vi "DIFFERENT OPERATIONS ON VALUES.vi"() -> ()   [LabVIEW 2015]
panel:
  in  "CHOOSE THE OPERATION":T1(ring)
  out "OUTPUT":dbl
  in  "NUM 2":dbl
  in  "NUM 1":dbl
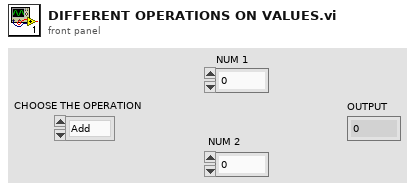
[diagram p1: front panel]
types:
  T1 = enum16{"Add", "Subtract", "Multiply", "Divide", "Max", "Min", "square", "sqrt", "avg"}
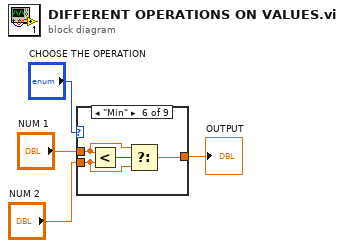
[diagram p0: block diagram]
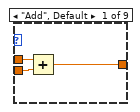
[diagram p2: hidden frame]
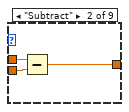
[diagram p3: hidden frame]
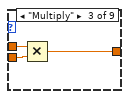
[diagram p4: hidden frame]
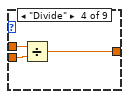
[diagram p5: hidden frame]
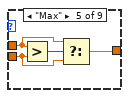
[diagram p6: hidden frame]
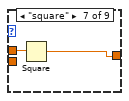
[diagram p7: hidden frame]
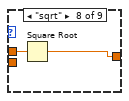
[diagram p8: hidden frame]
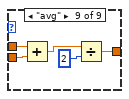
[diagram p9: hidden frame]
diagram:
  n1 = case shown="\"Min\"" "CHOOSE THE OPERATION" {
    tunnel: "NUM 1" -> [w7 w10 w13 w16 w19 w22 w26 w28 w33]
    tunnel: "NUM 2" -> [w6 w9 w12 w15 w18 w24 _ _ w32]
    tunnel: [w5 w8 w11 w14 w17 w21 w25 w27 w30] -> w1
    frame "Add", Default {
      n2 = Add(x=w7, y=w6) -> (x+y=w5:dbl)
    }
    frame "Subtract" {
      n3 = Subtract(x=w10, y=w9) -> (x-y=w8:dbl)
    }
    frame "Multiply" {
      n4 = Multiply(x=w13, y=w12) -> (x*y=w11:dbl)
    }
    frame "Divide" {
      n5 = Divide(x=w16, y=w15) -> (x/y=w14:dbl)
    }
    frame "Max" {
      n6 = Greater?(x=w19, y=w18) -> (0:w20:bool)
      n7 = Select(t=w19, s=w20, f=w18) -> (s? t:f=w17:dbl)
    }
    frame "Min" {
      n8 = Less?(x=w22, y=w24) -> (x < y?=w23:bool)
      n9 = Select(t=w22, s=w23, f=w24) -> (s? t:f=w21:dbl)
    }
    frame "square" {
      n10 = Square(x=w26) -> (x^2=w25:dbl)
    }
    frame "sqrt" {
      n11 = Square Root(x=w28) -> (sqrt(x)=w27:dbl)
    }
    frame "avg" {
      n12 = Add(x=w33, y=w32) -> (x+y=w31:dbl)
      n13 = Divide(x=w31, y=2) -> (x/y=w30:dbl)
    }
  }
  "OUTPUT" <- w1
